vi "ModularClient.vi"() -> ()   [LabVIEW 2013]
uses:
  Controls/SM States.ctl
  <vilib>/Instr/_visa.llb/VISA Configure Serial Port (Instr).vi
panel:
  in  "Submit":bool
  in  "Command":string="?"
  out "Response":string
  out "Msg":string
  in  "Methods":u16(ring)
  in  "Stop Button":bool
  in  "PORT ID":refnum<visa-resource-name>
  # "Modular Client"
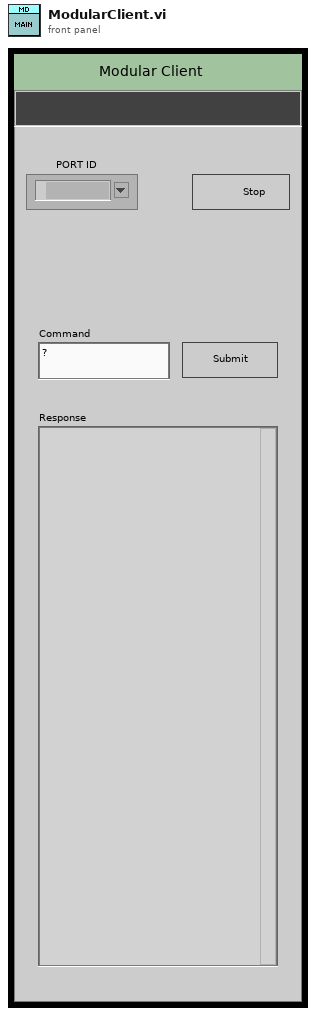
[diagram p1: front panel]
types:
  T1 = typedef "SM States.ctl" = enum16{"Connect to Device", "Get Methods", "Set Method", "Test", "STOP"}
  T2 = enum8{"Enabled", "Disabled", "Disabled and Grayed Out"}
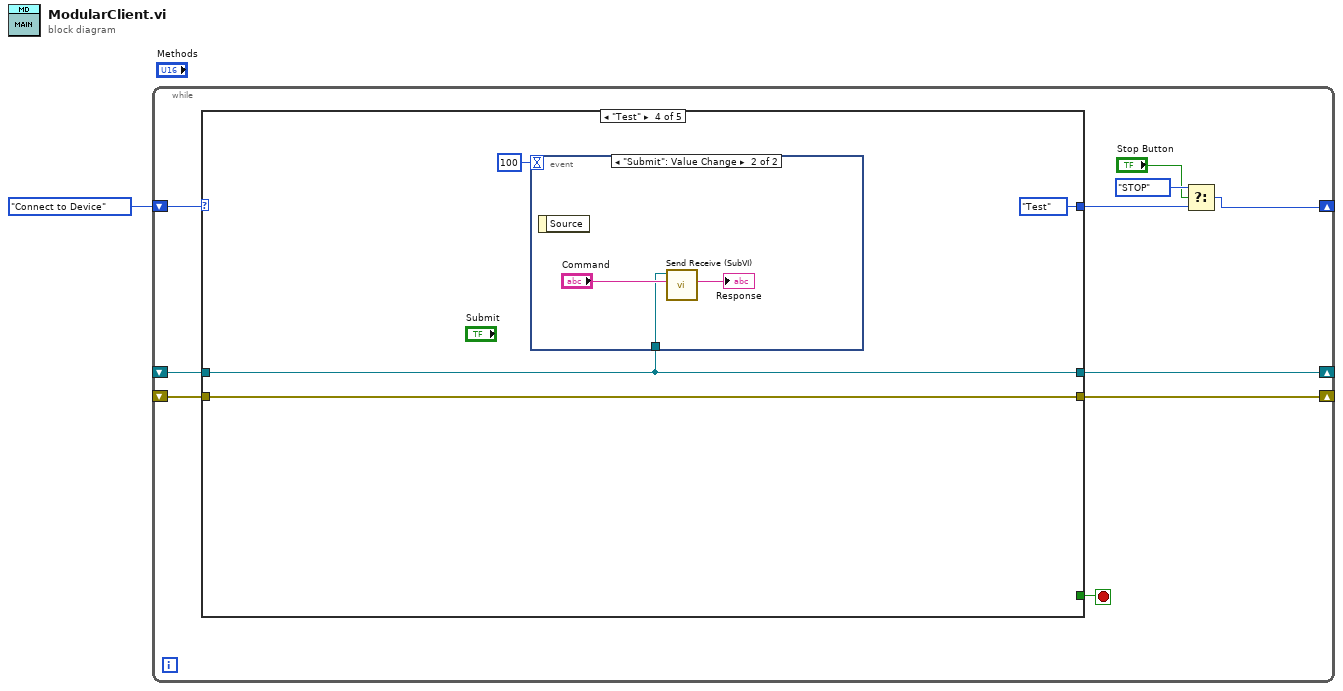
[diagram p0: block diagram]
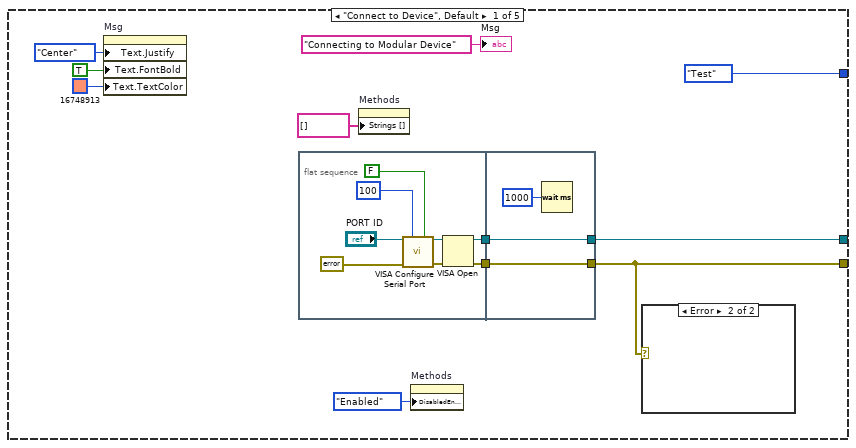
[diagram p2: hidden frame]
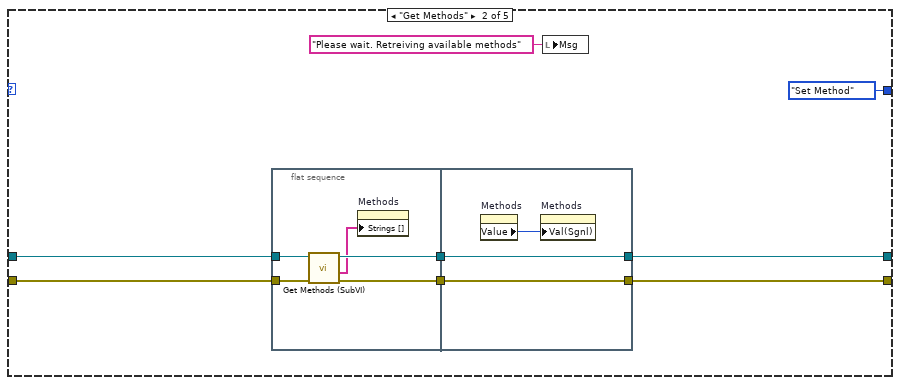
[diagram p4: hidden frame]
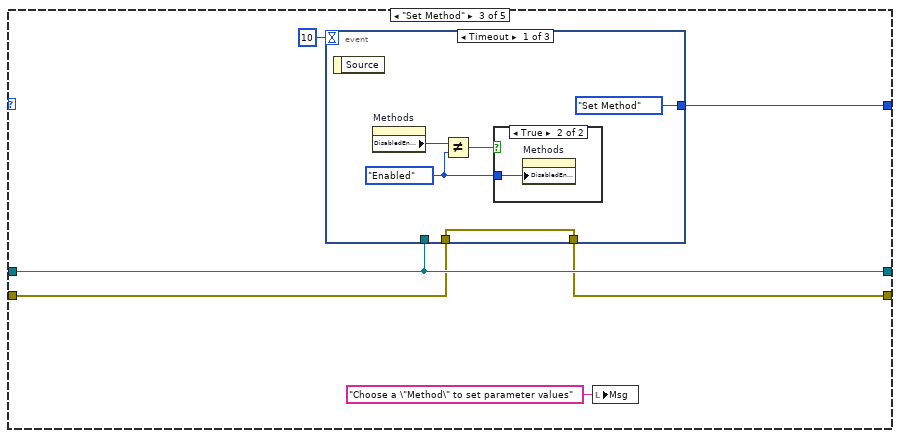
[diagram p5: hidden frame]
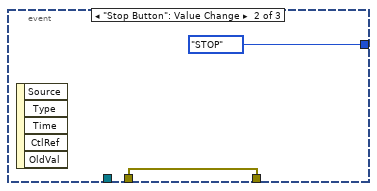
[diagram p7: hidden frame]
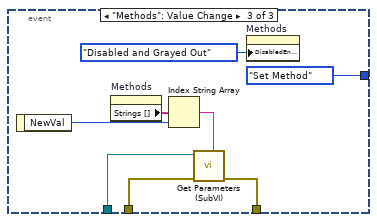
[diagram p8: hidden frame]
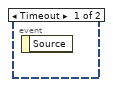
[diagram p9: hidden frame]
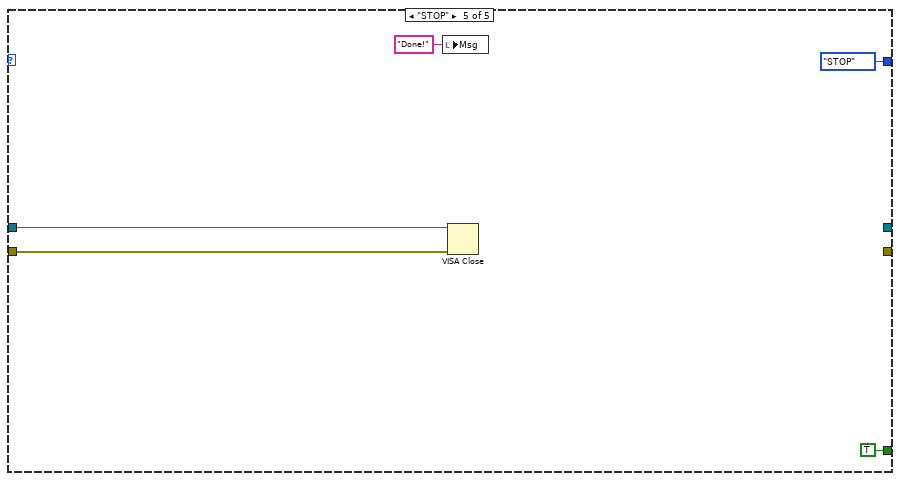
[diagram p10: hidden frame]
diagram:
  n1 = while {
    shift-right: [w5] -> _
    shift-left: SM_States."Connect to Device" -> [w11]
    shift-right: [w10] -> _
    shift-left: _ -> [w8]
    shift-right: [w9] -> _
    shift-left: _ -> [w7]
    stop <- w2 stop-if-true
    n2 = case shown="\"Test\"" w11 {
      tunnel: [w20 w41 w53 w72 _] -> w10
      tunnel: [w17 w40 w51 w74 _] -> w9
      tunnel: w8 -> [_ w39 w53 w72 w82]
      tunnel: w7 -> [_ w38 w52 w74 w83]
      tunnel: [SM_States."Test" SM_States."Set Method" w54 SM_States."Test" SM_States."STOP"] -> w6
      tunnel: [_ _ _ _ TRUE] -> w2
      frame "Connect to Device", Default {
        n3 = property on="Msg" class="Str"("Text.Justify"=enum16{"Left", "Center", "Right"}."Center" ("Text.Justification"), "Text.FontBold"=TRUE ("Text.Font:Bold"), "Text.TextColor"=u32 16748913) -> ()  [unwired: 2 in, 2 out]
        n4 = flat-sequence {
          tunnel: [w27] -> w22
          tunnel: [w25] -> w21
          tunnel: w22 -> [w33]
          tunnel: w21 -> [w32]
          tunnel: [w33] -> w20
          tunnel: [w32] -> w17
          frame #0 {
            n5 = call-poly "VISA Configure Serial Port"("VISA resource name"="PORT ID", "timeout (10sec)"=u32 100, "Enable Termination\nChar (T)"=FALSE ("Enable Termination\nChar (T)"), "error in (no error)"=errorcluster {"status"=FALSE, "code"=0, "source"=""}) -> ("VISA resource name out"=w29:refnum<visa-resource-name>, "error out"=w26:errorcluster)  [unwired: 10 in]
            n6 = VISA Open(error in (no error)=w26, VISA resource name=w29) -> (VISA resource name=w27:refnum<visa-resource-name>, error out=w25:errorcluster)  [unwired: 3 in]
          }
          frame #1 {
            n7 = Wait (ms)(milliseconds to wait=u32 1000) -> ()  [unwired: 1 out]
          }
        }
        n8 = property on="Methods" class="Ring (strict)"("Strings []"=string[] []) -> ()  [unwired: 2 in, 2 out]
        n9 = property on="Methods" class="Ring (strict)"("DisabledEnum"=T2."Enabled" ("Disabled")) -> ()  [unwired: 2 in, 2 out]
        n10 = case shown="Error" w17 {
          frame No Error {
          }
          frame Error {
          }
        }
        "Msg" <- "Connecting to Modular Device" ("Msg")
      }
      frame "Get Methods" {
        n11 = flat-sequence {
          tunnel: w39 -> [w44]
          tunnel: w38 -> [w43]
          tunnel: [w46] -> w35
          tunnel: [w45] -> w34
          tunnel: [w48] -> w40
          tunnel: [w49] -> w41
          tunnel: w35 -> [w49]
          tunnel: w34 -> [w48]
          frame #0 {
            n12 = call "Get Methods (SubVI).vi"("error in (no error)"=w43, "VISA Refnum in"=w44) -> ("error out"=w45:errorcluster, "Array"=w42:string[], "VISA Refnum out"=w46:refnum<visa-resource-name>)  [unwired: 6 in, 1 out]
            n13 = property on="Methods" class="Ring (strict)"("Strings []"=w42) -> ()  [unwired: 2 in, 2 out]
          }
          frame #1 {
            n14 = property on="Methods" class="Ring (strict)"() -> ("Value"=w47:u16)  [unwired: 2 in, 2 out]
            n15 = property on="Methods" class="Ring (strict)"("Val(Sgnl)"=w47) -> ()  [unwired: 2 in, 2 out]
          }
        }
        n16 = local write "Msg"("Please wait. Retreiving available methods" ("Msg")) -> ()
      }
      frame "Set Method" {
        n17 = event shown="[0] Timeout" {
          selector: _ -> [_ _ _]
          dyn-events: _ -> [_ _ _]
          timeout: 10 -> [_ _ _]
          tunnel: [SM_States."Set Method" SM_States."STOP" SM_States."Set Method"] -> w54
          tunnel: w53 -> [_ _ w68]
          tunnel: w52 -> [w59 w62 w67]
          tunnel: [w59 w62 w65] -> w51
          event Timeout {
            w57 = T2."Enabled" ("Disabled")
            n18 = event-data() -> ()  [unwired: 1 in, 1 out]
            n19 = property on="Methods" class="Ring (strict)"() -> ("DisabledEnum"=w58:T2)  [unwired: 2 in, 2 out]
            n20 = Not Equal?(x=w58, y=w57) -> (x != y?=w56:bool)
            n21 = case shown="True" w56 {
              tunnel: w57 -> [_ w61]
              frame False {
              }
              frame True {
                n22 = property on="Methods" class="Ring (strict)"("DisabledEnum"=w61) -> ()  [unwired: 2 in, 2 out]
              }
            }
          }
          event "Stop Button": Value Change {
            n23 = event-data() -> ()  [unwired: 1 in, 5 out]
          }
          event "Methods": Value Change {
            n24 = event-data() -> ("NewVal"=w70:u16)  [unwired: 1 in]
            n25 = property on="Methods" class="Ring (strict)"() -> ("Strings []"=w71:string[])  [unwired: 2 in, 2 out]
            n26 = Index String Array(1:w70, 2:w71) -> (0:w66:string)  [unwired: 1 in]
            n27 = call "Get Parameters (SubVI).vi"("Command"=w66, "error in (no error)"=w67, "VISA Refnum in"=w68) -> ("error out"=w65:errorcluster)  [unwired: 5 in, 3 out]
            n28 = property on="Methods" class="Ring (strict)"("DisabledEnum"=T2."Disabled and Grayed Out" ("Disabled")) -> ()  [unwired: 2 in, 2 out]
          }
        }
        n29 = local write "Msg"("Choose a \"Method\" to set parameter values" ("Msg")) -> ()
      }
      frame "Test" {
        n30 = event shown="[1] \"Submit\": Value Change" {
          selector: _ -> [_ _]
          dyn-events: _ -> [_ _]
          timeout: 100 -> [_ _]
          tunnel: w72 -> [_ w76]
          event Timeout {
            n31 = event-data() -> ()  [unwired: 1 in, 1 out]
          }
          event "Submit": Value Change {
            n32 = event-data() -> ()  [unwired: 1 in, 1 out]
            n33 = call "Send Receive (SubVI).vi"("Command"="Command", "VISA Refnum in"=w76) -> ("Response"=→"Response":string)  [unwired: 7 in, 2 out]
          }
        }
      }
      frame "STOP" {
        n34 = local write "Msg"("Done!" ("Msg")) -> ()
        n35 = VISA Close(VISA resource name=w82, error in (no error)=w83) -> ()  [unwired: 1 out]
      }
    }
    n36 = Select(t=SM_States."STOP", s="Stop Button", f=w6) -> (s? t:f=w5:T1)
  }
